vi "energy_detection2.vi"() -> ()   [LabVIEW 2014]
uses:
  <vilib>/Analysis/2dsp.llb/Complex FFT.vi
  <vilib>/Analysis/7linalg.llb/Complex Eigenvalues and Vectors.vi
  Comm_Lab_Final/var_stop.vi
  <vilib>/Analysis/7linalg.llb/Create Special Real Matrix.vi
  <vilib>/Analysis/Matrix/Numeric/Conversions/Matrix To Array - RM.vi
  <vilib>/Analysis/Matrix/Numeric/Multiply/Multiply - RM,R.vi
  <instrlib>/niUSRP/niUSRP Fetch Rx Data (CDB Cluster).vi
  <vilib>/Analysis/2dsp.llb/AutoCorrelation Matrix (CDB).vi
  <vilib>/Analysis/Matrix/Numeric/Conversions/Matrix To Array - CM.vi
  <vilib>/measure/maspectr.llb/FFT Power Spectrum and PSD for 1 Chan (CDB).vi
  <vilib>/measure/madcrms.llb/Averaged DC-RMS for 1 Chan.vi
  <vilib>/Analysis/NI_AAL_SigProc.lvlib
  <vilib>/Analysis/NI_AALPro.lvlib
  <vilib>/Analysis/Matrix/NI_Matrix.lvlib
  <vilib>/measure/NI_MAPro.lvlib
panel:
  out "Noise Average":dbl
  out "Signal Average":dbl
  in  "Average size":i32=10
  in  "Noise Threshold":dbl=-105.0 format="%#_6f"
  out "Average Noise floor in dBm per Hz":dbl
  out "Eigenvalues":cdb[](array[numeric]) format="%.2f"
  out "Real 2D Array":dbl[][](array[numeric])
  out "df":dbl
  out "f0":dbl
  out "Min Eigenvalue method":bool
  out "Minimum eigenvalue method":dbl
  out "Energy of the Signal":dbl
  out "min eigen value":dbl
  out "max eigen value":dbl
  out "my average power":dbl
  out "size(s)":i32
  out "Waveform Graph 2":dbl[](graph)
  out "Waveform Graph":dbl[](graph)
  out "Carrier Freq":dbl
  in  "stop":bool
  out "Power Spectrum / PSD":cluster{"f0":dbl, "df":dbl, "magnitude":dbl[]}(graph)
  out "data":waveform(cdb)
  in  "timeout":dbl=10.0
  in  "number of samples":i64=100000
  out "coerced gain":dbl format="%#_6f"
  out "Noise floor in dBm per Hz":dbl
  in  "matrix type(Dont Change), need to be indentity":i32
  in  "order of AC matrix":i32=8
  out "Energy of the Signal in dBm per Hz":dbl
  out "coerced carrier frequency":dbl format="%#_6p"
  out "coerced IQ rate":dbl format="%#_6p"
  in  "gain":dbl format="%#_6f"
  in  "IQ rate":dbl=800000.0 format="%#_6p"
  in  "RX device names":refnum<k15>="192.168.10.3"
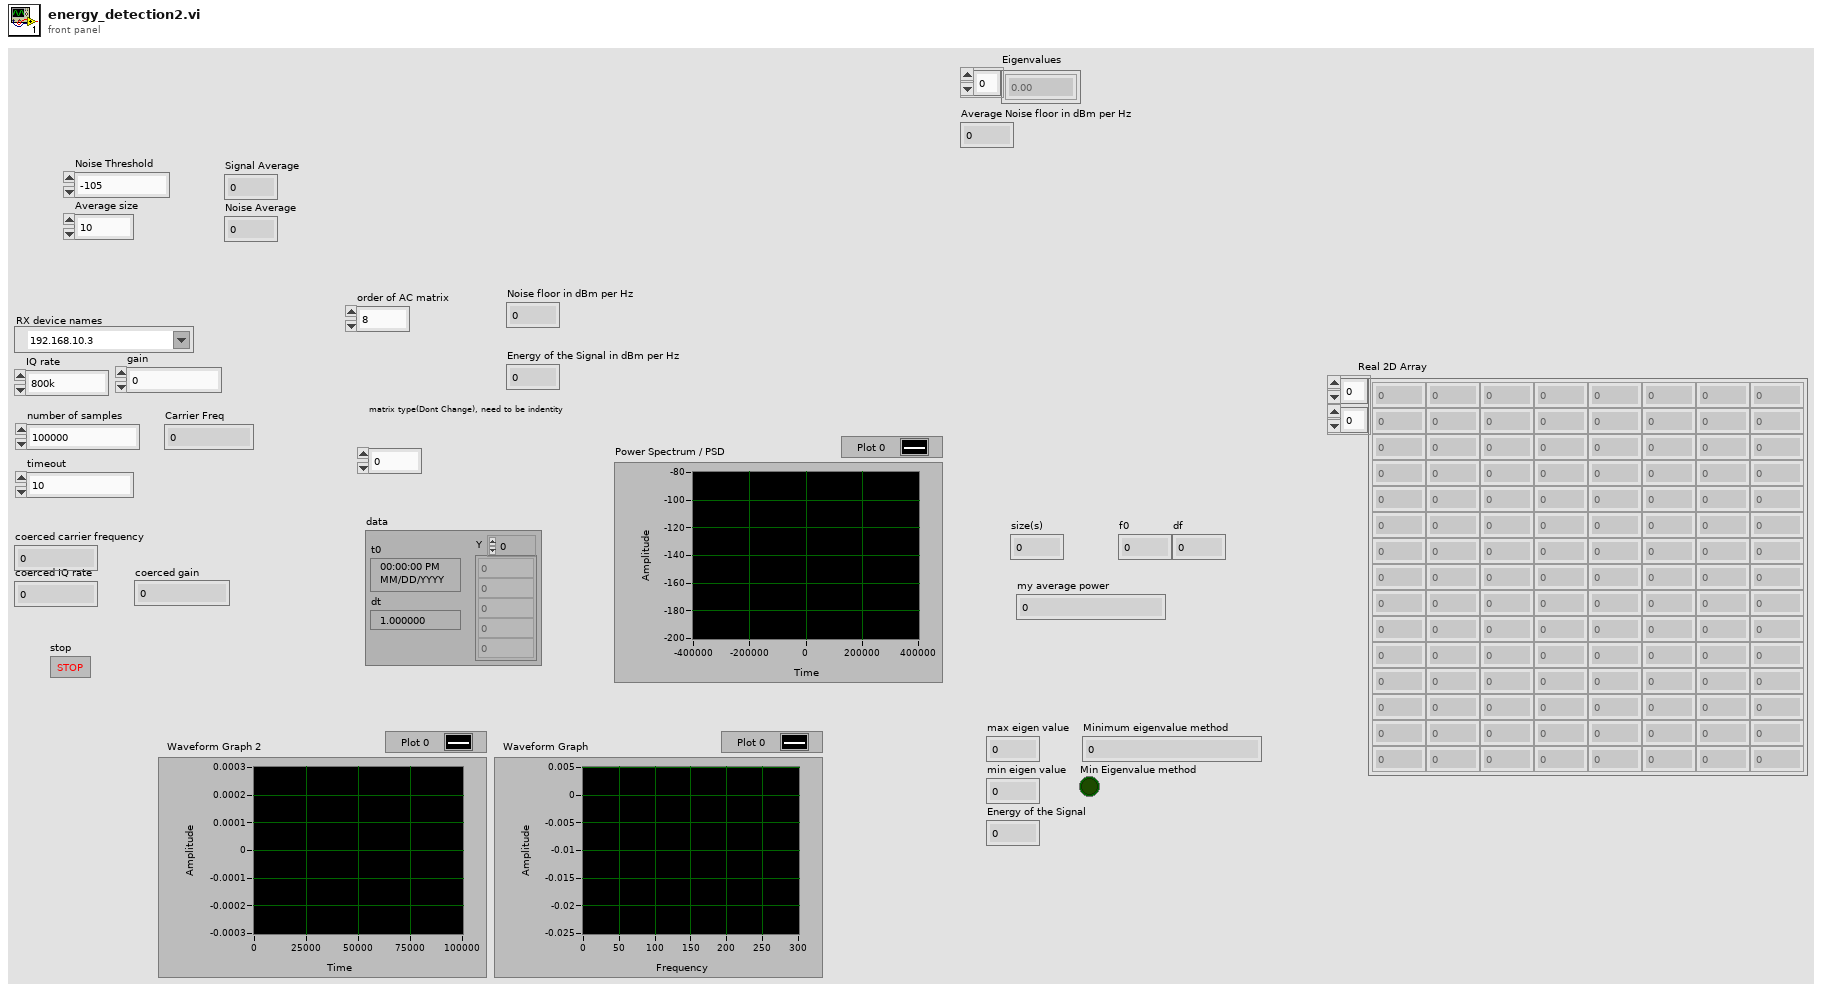
[diagram p1: front panel]
types:
  T1 = typedef "NI_Matrix.lvlib/RealMatrix.ctl" = dbl[][]
  T2 = typedef "NI_Matrix.lvlib/ComplexMatrix.ctl" = cdb[][]
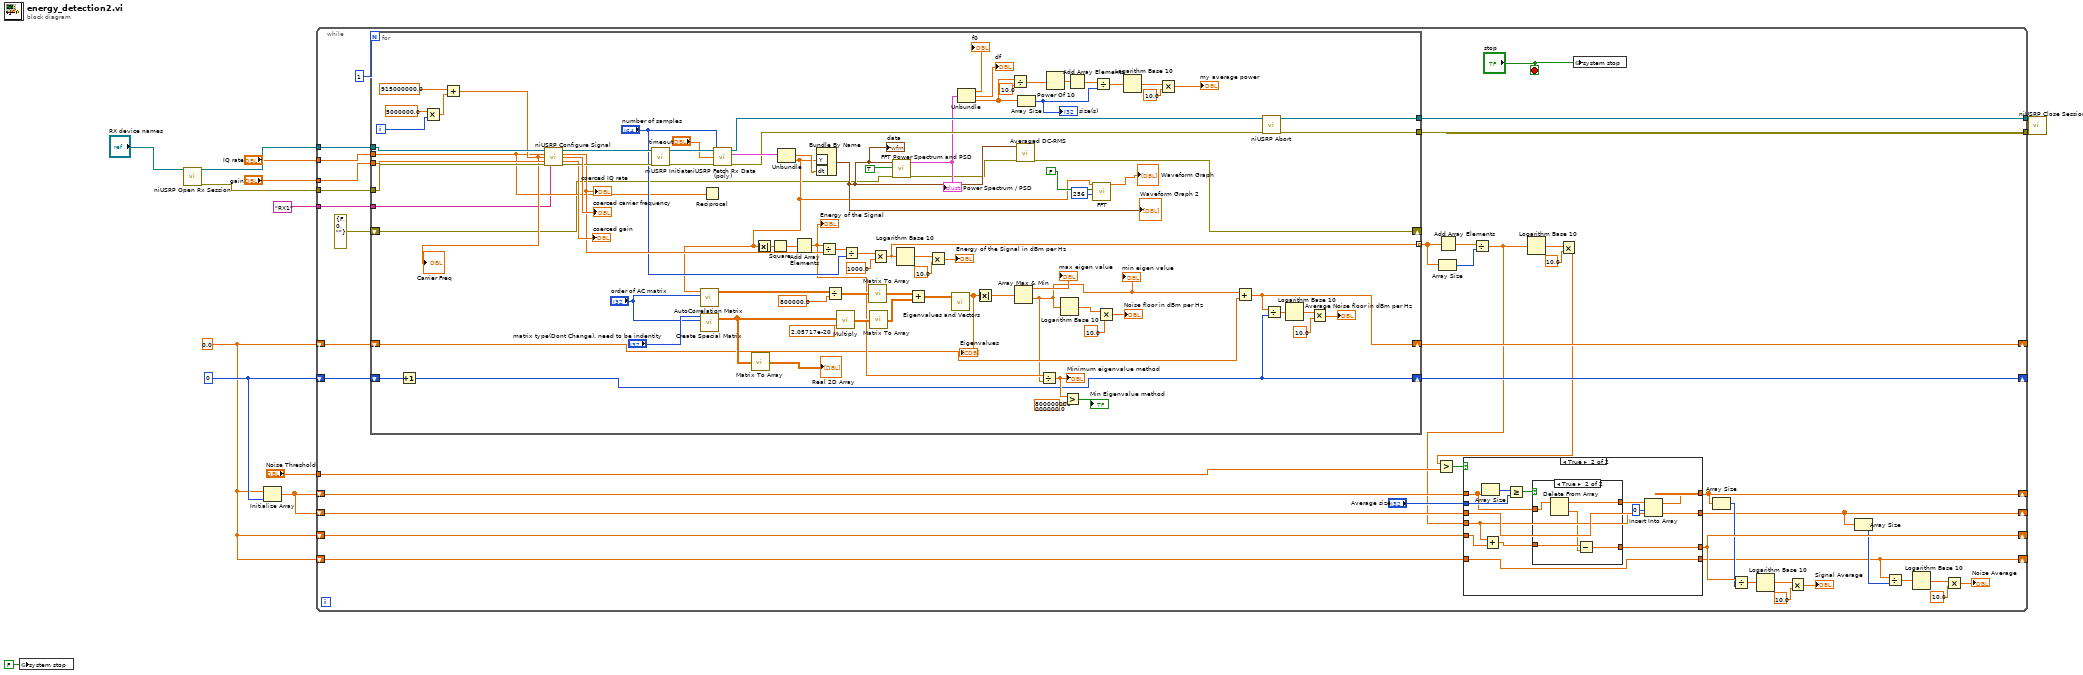
[diagram p0: block diagram]
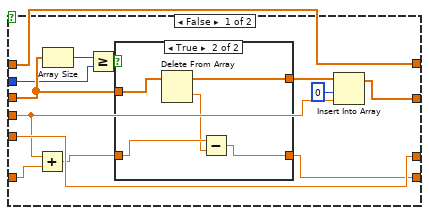
[diagram p2: hidden frame]
diagram:
  w1 = 0.0
  w4 = 0
  n1 = global write "var_stop.vi" "system stop"(FALSE) -> ()
  n2 = call <instrlib>:"niUSRP Open Rx Session.vi"("device names"="RX device names") -> ("session handle out"=w11:refnum<k15>, "error out"=w10:errorcluster)  [unwired: 13 in]
  n3 = Initialize Array(w1, w4) -> (w3:dbl[])
  n4 = while {
    tunnel: w11 -> [w51]
    tunnel: w10 -> [w54]
    tunnel: "IQ rate" -> [w53]
    tunnel: "gain" -> [w52]
    tunnel: [w50] -> w7
    tunnel: [w49] -> w6
    tunnel: "RX1" ("active antenna") -> [w48]
    shift-right: [w43] -> _
    shift-left: w4 -> [w46]
    shift-right: [w44] -> _
    shift-left: w1 -> [w45]
    shift-right: [w17] -> _
    shift-left: w3 -> [w34]
    shift-right: [w20] -> _
    shift-left: w3 -> [w35]
    tunnel: "Noise Threshold" -> [w37]
    shift-right: [w21] -> _
    shift-left: w1 -> [w32]
    shift-right: [w16] -> _
    shift-left: w1 -> [w31]
    stop <- "stop" stop-if-true
    n5 = for {
      N: 1 -> [_]
      tunnel: w54 -> [w173]
      tunnel: w53 -> [w139]
      tunnel: w52 -> [w172]
      tunnel: w51 -> [w171]
      tunnel: [w142] -> w50
      tunnel: [w141] -> w49
      tunnel: w48 -> [w138]
      shift-right: [w111] -> _
      shift-left: errorcluster {"status"=FALSE, "code"=0, "source"=""} ("error out") -> [w113]
      shift-right: [w104] -> w43
      shift-left: w46 -> [w107]
      shift-right: [w105] -> w44
      shift-left: w45 -> [w106]
      tunnel: [w97] -> w42 mode=indexing
      i -> [w181]
      n6 = Increment(x=w107) -> (x+1=w104:i32)
      n7 = Multiply(x=5000000.0, y=w181) -> (x*y=w179:dbl)
      n8 = Add(x=915000000.0, y=w179) -> (x+y=w140:dbl)
      "Carrier Freq" <- w140
      n9 = call <instrlib>:"niUSRP Configure Signal.vi"("session handle"=w171, "IQ rate"=w139, "carrier frequency"=w140, "gain"=w172, "error in (no error)"=w173, "active antenna"=w138) -> ("session handle out"=w177:refnum<k15>, "coerced IQ rate"=w146:dbl, "coerced carrier frequency"=→"coerced carrier frequency":dbl, "coerced gain"=→"coerced gain":dbl, "error out"=w176:errorcluster)  [unwired: 5 in]
      "coerced IQ rate" <- w146
      n10 = call <instrlib>:"niUSRP Initiate.vi"("session handle"=w177, "error in (no error)"=w176) -> ("session handle out"=w175:refnum<k15>, "error out"=w174:errorcluster)  [unwired: 12 in]
      n11 = call-poly <vilib>:"Create Special Matrix.vi"("matrix type"="matrix type(Dont Change), need to be indentity", "matrix size"="order of AC matrix") -> ("Special Matrix"=w110:T1)  [unwired: 3 in, 1 out]
      n12 = Reciprocal(x=w139) -> ()  [unwired: 1 out]
      n13 = call-poly <instrlib>:"niUSRP Fetch Rx Data (poly).vi"("session handle"=w175, "number of samples"="number of samples", "timeout"="timeout", "error in (no error)"=w174) -> ("session handle out"=w143:refnum<k15>, "data"=w147:cluster{"t0":dbl, "dt":dbl, "Y":cdb[]}, "error out"=w144:errorcluster)  [unwired: 8 in, 1 out]
      n14 = call-poly <vilib>:"Matrix To Array.vi"("Real Matrix"=w110) -> ("Real 2D Array"=→"Real 2D Array":dbl[][])
      n15 = Unbundle(w147) -> ("dt"=w137:dbl, "Y"=w132:cdb[])  [unwired: 1 out]
      n16 = call-poly <vilib>:"AutoCorrelation Matrix.vi"("order"="order of AC matrix", "X"=w132) -> ("AutoCorrelation Matrix"=w154:T2)  [unwired: 8 in, 1 out]
      n17 = Absolute Value(x=w132) -> (abs(x)=w96:dbl[])
      n18 = Square(x=w96) -> (x^2=w149:dbl[])
      n19 = Add Array Elements(numeric array=w149) -> (sum=w127:dbl)
      "Energy of the Signal" <- w127
      n20 = Bundle By Name("Y"=w132, "dt"=w137) -> (w134:waveform(cdb))  [unwired: 1 in]
      "data" <- w134
      "Waveform Graph 2" <- w134
      n21 = Divide(x=w127, y=w146) -> (x/y=w167:dbl)
      n22 = Divide(x=w154, y=800000.0) -> (x/y=w159:T2)
      n23 = call-poly <vilib>:"Multiply.vi"("Real Scalar c"=2.05717e-20, "Real Matrix A"=w110) -> ("A * c"=w160:T1)
      n24 = Divide(x=w167, y="number of samples") -> (x/y=w98:dbl)
      n25 = call-poly <vilib>:"Matrix To Array.vi"("Complex Matrix"=w159) -> ("Complex 2D Array"=w161:cdb[][])
      n26 = call-poly <vilib>:"Matrix To Array.vi"("Real Matrix"=w160) -> ("Real 2D Array"=w162:dbl[][])
      n27 = Multiply(x=w98, y=1000.0) -> (x*y=w97:dbl)
      n28 = call-poly <vilib>:"FFT Power Spectrum and PSD.vi"("error in (no error)"=w113, "dB On (F)"=TRUE ("reset? (T)"), "time signal"=w134) -> ("error out"=w112:errorcluster, "Power Spectrum / PSD"=w131:cluster{"f0":dbl, "df":dbl, "magnitude":dbl[]})  [unwired: 5 in, 2 out]
      "Power Spectrum / PSD" <- w131
      n29 = Logarithm Base 10(1:w97) -> (0:w151:dbl)
      n30 = Add(x=w161, y=w162) -> (x+y=w163:cdb[][])
      n31 = Multiply(x=w151, y=10.0) -> (x*y=→"Energy of the Signal in dBm per Hz":dbl)
      n32 = call-poly <vilib>:"Eigenvalues and Vectors.vi"("Input Matrix"=w163) -> ("Eigenvalues"=w164:cdb[])  [unwired: 2 in, 2 out]
      "Eigenvalues" <- w164
      n33 = Unbundle(w131) -> ("f0"=→"f0":dbl, "df"=→"df":dbl, "magnitude"=w120:dbl[])
      n34 = Absolute Value(x=w164) -> (abs(x)=w168:dbl[])
      n35 = Divide(x=w120, y=10.0) -> (x/y=w121:dbl[])
      n36 = Array Max & Min(array=w168) -> (max value=→"max eigen value":dbl, min value=w103:dbl)  [unwired: 2 out]
      "min eigen value" <- w103
      n37 = call-poly <vilib>:"Averaged DC-RMS.vi"("error in (no error)"=w112, "signal in"=w134) -> ("error out"=w111:errorcluster)  [unwired: 5 in, 4 out]
      n38 = Array Size(array=w120) -> (size(s)=w129:i32)
      "size(s)" <- w129
      n39 = Divide(x=w127, y=w103) -> (x/y=w126:dbl)
      "Minimum eigenvalue method" <- w126
      n40 = Power Of 10(x=w121) -> (10^x=w118:dbl[])
      n41 = Logarithm Base 10(1:w103) -> (0:w165:dbl)
      n42 = Greater?(x=w126, y=800000000000000.0) -> (0:→"Min Eigenvalue method":bool)
      n43 = Add Array Elements(numeric array=w118) -> (sum=w130:dbl)
      n44 = call-poly <vilib>:"FFT.vi"("FFT size"=256, "shift?"=FALSE, "X"=w132) -> ("FFT {X}"=→"Waveform Graph":cdb[])  [unwired: 7 in, 1 out]
      n45 = Divide(x=w130, y=w129) -> (x/y=w117:dbl)
      n46 = Multiply(x=w165, y=10.0) -> (x*y=→"Noise floor in dBm per Hz":dbl)
      n47 = Logarithm Base 10(1:w117) -> (0:w116:dbl)
      n48 = Multiply(x=w116, y=10.0) -> (x*y=→"my average power":dbl)
      n49 = Add(x=w103, y=w106) -> (x+y=w105:dbl)
      n50 = call <instrlib>:"niUSRP Abort.vi"("session handle"=w143, "error in (no error)"=w144) -> ("session handle out"=w142:refnum<k15>, "error out"=w141:errorcluster)  [unwired: 12 in]
      n51 = Divide(x=w105, y=w104) -> (x/y=w102:dbl)
      n52 = Logarithm Base 10(1:w102) -> (0:w101:dbl)
      n53 = Multiply(x=w101, y=10.0) -> (x*y=→"Average Noise floor in dBm per Hz":dbl)
    }
    n54 = Array Size(array=w42) -> (size(s)=w40:i32)
    n55 = Add Array Elements(numeric array=w42) -> (sum=w41:dbl)
    n56 = Divide(x=w41, y=w40) -> (x/y=w24:dbl)
    n57 = Logarithm Base 10(1:w24) -> (0:w25:dbl)
    n58 = Multiply(x=w25, y=10.0) -> (x*y=w23:dbl)
    n59 = Greater?(x=w23, y=w37) -> (0:w36:bool)
    n60 = case shown="True" w36 {
      tunnel: w35 -> [w62 w85]
      tunnel: w34 -> [w64 w81]
      tunnel: "Average size" -> [w63 w87]
      tunnel: w24 -> [w57 w78]
      tunnel: [w62 w82] -> w20
      tunnel: [w61 w81] -> w17
      tunnel: w32 -> [w60 w77]
      tunnel: w31 -> [w58 w80]
      tunnel: [w59 w80] -> w16
      tunnel: [w60 w79] -> w21
      frame False {
        n61 = Add(x=w57, y=w58) -> (x+y=w56:dbl)
        n62 = Array Size(array=w64) -> (size(s)=w65:i32)
        n63 = Greater Or Equal?(x=w65, y=w63) -> (x >= y?=w66:bool)
        n64 = case shown="True" w66 {
          tunnel: w64 -> [w70 w75]
          tunnel: [w70 w74] -> w67
          tunnel: w56 -> [w69 w73]
          tunnel: [w69 w71] -> w59
          frame False {
          }
          frame True {
            n65 = Delete From Array(array=w75) -> (deleted portion=w72:dbl, array with subset deleted=w74:dbl[])  [unwired: 2 in]
            n66 = Subtract(x=w73, y=w72) -> (x-y=w71:dbl)
          }
        }
        n67 = Insert Into Array(array=w67, index=0, new element=w57) -> (w61:dbl[])
      }
      frame True {
        n68 = Array Size(array=w85) -> (size(s)=w88:i32)
        n69 = Add(x=w78, y=w77) -> (x+y=w76:dbl)
        n70 = Greater Or Equal?(x=w88, y=w87) -> (x >= y?=w86:bool)
        n71 = case shown="True" w86 {
          tunnel: w85 -> [w90 w95]
          tunnel: [w90 w94] -> w84
          tunnel: w76 -> [w89 w93]
          tunnel: [w89 w91] -> w79
          frame False {
          }
          frame True {
            n72 = Delete From Array(array=w95) -> (deleted portion=w92:dbl, array with subset deleted=w94:dbl[])  [unwired: 2 in]
            n73 = Subtract(x=w93, y=w92) -> (x-y=w91:dbl)
          }
        }
        n74 = Insert Into Array(array=w84, index=0, new element=w78) -> (w82:dbl[])
      }
    }
    n75 = global write "var_stop.vi" "system stop"("stop") -> ()
    n76 = Array Size(array=w20) -> (size(s)=w19:i32)
    n77 = Divide(x=w21, y=w19) -> (x/y=w22:dbl)
    n78 = Logarithm Base 10(1:w22) -> (0:w38:dbl)
    n79 = Multiply(x=w38, y=10.0) -> (x*y=→"Signal Average":dbl)
    n80 = Array Size(array=w17) -> (size(s)=w18:i32)
    n81 = Divide(x=w16, y=w18) -> (x/y=w15:dbl)
    n82 = Logarithm Base 10(1:w15) -> (0:w28:dbl)
    n83 = Multiply(x=w28, y=10.0) -> (x*y=→"Noise Average":dbl)
  }
  n84 = call <instrlib>:"niUSRP Close Session.vi"("session handle"=w7, "error in (no error)"=w6) -> ()  [unwired: 13 in, 1 out]
